vi "IMAQ FPGA Configure Image Transfer from Target U16.vi"(5 "DMA FIFO Depth in Images":u32=2, 7 "Image Size":T1, 8 "error in (no error)":errorcluster, 9 "DMA FIFO Name":string, 10 "FPGA VI Reference In":refnum<k20>, 11 "Image":T2) -> (0 "error out":errorcluster, 1 "DMA FIFO Reference Out":refnum<k20>, 3 "Image Out":T2)   [LabVIEW 2017, in "NI_VDM_FPGA_Basics.lvlib"]
doc: "Configures the transfer of an image from the target FPGA to the host processor via a DMA FIFO. If the <B>Image Size</B> control specifies non-zero <B>Width</B> and <B>Height</B> values, then the image referenced by Image will be resized to match those values. Otherwise, the original image size is preserved. In addition, a reference will be opened to the DMA FIFO that will be used to transfer the image from the target FPGA to the host computer."
uses:
  <vilib>/visionFPGA/NI_VDM_FPGA_Basics.lvlib
  <vilib>/vision/Image Controls.llb/IMAQ Image.ctl
  <vilib>/visionFPGA/Controls/IMAQ FPGA Image Size.ctl
  <vilib>/NI/LVFPGA Adv Session Resources/OpenByNameSubVI.vi
  <vilib>/Utility/error.llb/Error Cluster From Error Code.vi
  <vilib>/rvi/interface/common/niFpgaWaitOnOcc.vi
  <vilib>/rvi/interface/common/dynamic/niFpgaEscapeDelimiterAndNull.vi
  <vilib>/rvi/interface/nirviMethod/nirviMethod.xnode
  <vilib>/NI/LVFPGA Adv Session Resources/OpenByName.xnode
  <vilib>/rvi/errors/niLvFpgaMergeErrorWithErrorCode.vi
  <vilib>/FPGAPlugInAG/Dynamic/niLvFpga_ConfigureFifo_Dynamic.vi
  <vilib>/FPGAPlugInAG/Dynamic/niLvFpga_StartFifo_Dynamic.vi
  <vilib>/NI/LVFPGA Adv Session Resources/LVFPGAAdvSessionResources.lvlib
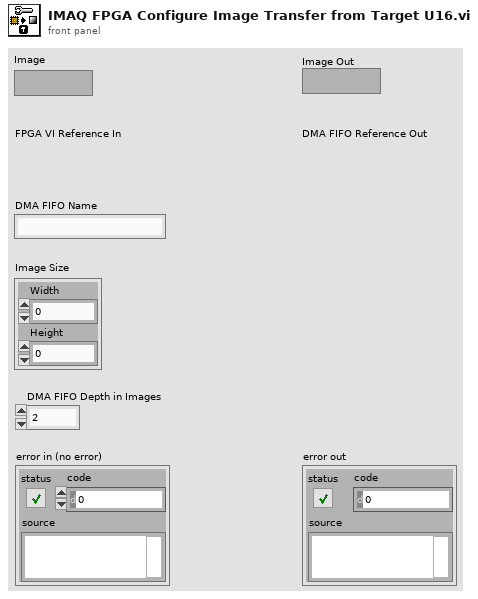
[diagram p1: front panel]
types:
  T1 = typedef "IMAQ FPGA Image Size.ctl" = cluster{"Width":u32, "Height":u32}
  T2 = typedef "IMAQ Image.ctl" = refnum<image>
  T3 = cluster{"Name":string, "Depth":u32, "Write? (Deprecated:Use Implementation)":bool, "Physical Channel":u32, "Base Address":u32, "Data Width":u32, "Data Type":enum32{"Boolean", "I8", "I16", "I32", "I64", "U8", "U16", "U32", "U64", "FXP", "CustomControl", "SGL"}, "FXP Properties":variant, "Write Window Address":u32, "Implementation":enum16{"niFpgaTargetToHost", "niFpgaHostToTarget", "niFpgaPeerToPeerWriter", "niFpgaPeerToPeerReader", "niCoreTargetToHost", "niCoreHostToTarget"}, "Control Set":u32}[]
  T4 = cluster{"Name":string, "type":variant, "indicator?":bool}[]
  T5 = typedef "Image Type" = u32
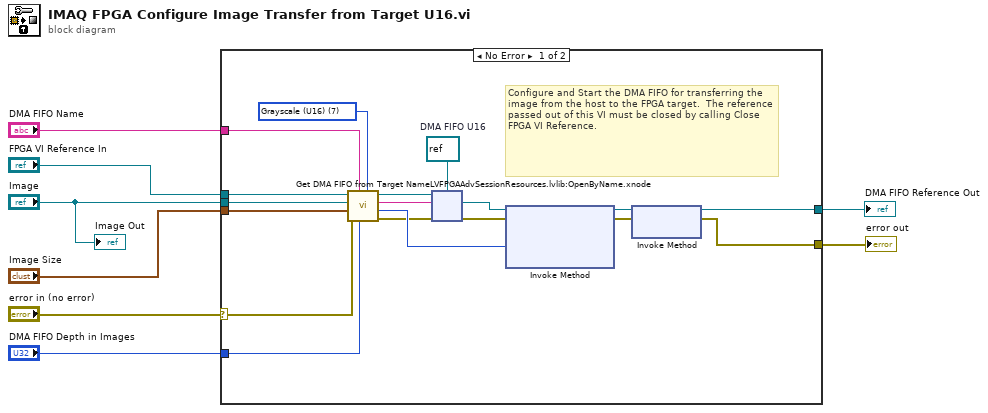
[diagram p0: block diagram]
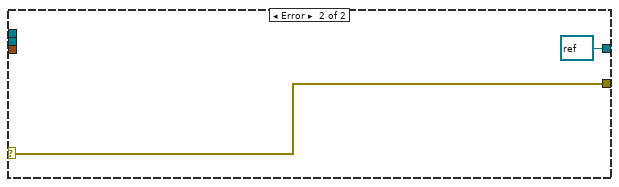
[diagram p2: hidden frame]
diagram:
  n1 = case shown="No Error" "error in (no error)" {
    selector: "error in (no error)" -> [w9 w41]
    tunnel: [w24 w41] -> w8
    tunnel: "DMA FIFO Depth in Images" -> [w23 _]
    tunnel: "FPGA VI Reference In" -> [w22 _]
    tunnel: "DMA FIFO Name" -> [w21 _]
    tunnel: "Image" -> [w20 _]
    tunnel: "Image Size" -> [w19 _]
    tunnel: [w16 refnum<k20> refnum ("FPGA VI Reference Out")] -> w2
    frame No Error {
      w15 = refnum<k20> refnum  # DMA FIFO U16
      w17 = T5 7 items=["Grayscale (U8)", "Grayscale (I16)", "Grayscale (SGL)", "Complex (CSG)", "RGB (U32)", "HSL (U32)", "RGB (U64)", "Grayscale (U16)"] ("Expected Image Type")
      # "Configure and Start the DMA FIFO for transferring the image from the host to the FPGA target.  The reference passed out of this VI must be closed by calling Close FPGA VI Reference."
      n2 = call <vilib>:"Get DMA FIFO from Target Name.vi"("Expected Image Type"=w17, "DMA FIFO Depth in Images"=w23, "DMA FIFO Name"=w21, "error in (no error)"=w9, "Image Size"=w19, "Image"=w20, "Refnum in"=w22) -> ("error out"=w14:errorcluster, "DMA FIFO Size"=w18:u32, "DMA FIFO from Target Name"=w11:string, "Refnum out"=w10:refnum<k20>)  [unwired: 1 in]
      n3 = xnode "LVFPGAAdvSessionResources.lvlib:OpenByName.xnode"("FPGA VI Reference in"=w10, "Resource name in"=w11, "Single resource reference type in"=w15, "Error in"=w14) -> ("Single resource reference out"=w12:refnum<k20>, "Error out"=w13:errorcluster)  [unwired: 1 out]
      n4 = xnode "Invoke Method"("FPGA VI Reference In"=w12, "error in"=w13, "Requested Depth"=w18) -> ("FPGA VI Reference Out"=w26:refnum<k20>, "error out"=w25:errorcluster)  [unwired: 1 out]
      n5 = xnode "Invoke Method"("FPGA VI Reference In"=w26, "error in"=w25) -> ("FPGA VI Reference Out"=w16:refnum<k20>, "error out"=w24:errorcluster)
    }
    frame Error {
    }
  }
  "error out" <- w8
  "DMA FIFO Reference Out" <- w2
  "Image Out" <- "Image"
